vi "SubVI_Amplifier_Setup_Impedances.vi"(8 "error in (no error)":errorcluster, 9 "LINX Resource in":T1, 10 "Command Row Lenghts":u8[](array[numeric]), 11 "Amplifier Commands":u8[][](array[numeric])) -> (0 "error out":errorcluster, 3 "LINX Resource out":T1)   [LabVIEW 2020]
uses:
  <vilib>/MakerHub/LINX/Private/Type Defs/LINX Ref.ctl
  <vilib>/MakerHub/LINX/Private/Type Defs/Platform.ctl
  <vilib>/MakerHub/LINX/Private/Type Defs/Interface.ctl
  <vilib>/MakerHub/LINX/Private/Device/Type Defs/LINX Device Config.ctl
  <vilib>/MakerHub/LINX/Private/Device/Type Defs/TCP Config.ctl
  <vilib>/MakerHub/LINX/Private/Device/Type Defs/Channels.ctl
  <vilib>/MakerHub/LINX/Private/Type Defs/Peripherals/SPI/SPI Configuration.ctl
  <vilib>/MakerHub/LINX/Private/Type Defs/Peripherals/SPI/SPI Bit Order.ctl
  <vilib>/MakerHub/LINX/Private/Type Defs/Peripherals/SPI/SPI Mode.ctl
  <vilib>/MakerHub/LINX/Public/Peripherals/SPI/SPI CS Config.ctl
  <vilib>/MakerHub/LINX/Private/Type Defs/Peripherals/SPI/SPI CS Logic Level.ctl
  <vilib>/MakerHub/LINX/Public/Peripherals/Digital/Digital Write 1 Chan.vi
  <vilib>/MakerHub/LINX/Public/Peripherals/Digital/Digital Read 1 Chan.vi
  <vilib>/MakerHub/LINX/Public/Peripherals/SPI/SPI Write Read N Frames.vi
  <vilib>/MakerHub/LINX/Public/Peripherals/Digital/Digital Write N Chans.vi
  <vilib>/MakerHub/LINX/Public/Peripherals/Digital/Digital Read N Chans.vi
  <vilib>/MakerHub/LINX/Private/Local IO/LinxSpiWriteRead.vi
  <vilib>/MakerHub/LINX/Public/Utilities/Check Channel.vi
  <vilib>/MakerHub/LINX/Private/Local IO/LinxDigitalWrite.vi
  <vilib>/MakerHub/LINX/Private/Local IO/LinxDigitalRead.vi
  <vilib>/MakerHub/LINX/Private/Local IO/Handle Errors.vi
  <vilib>/MakerHub/LINX/Private/Utilties/Generate Error.vi
  Global 1.vi
  <vilib>/MakerHub/LINX/LMH-LINX.lvlib
  <vilib>/MakerHub/LINX/Private/Device/Device.lvlib
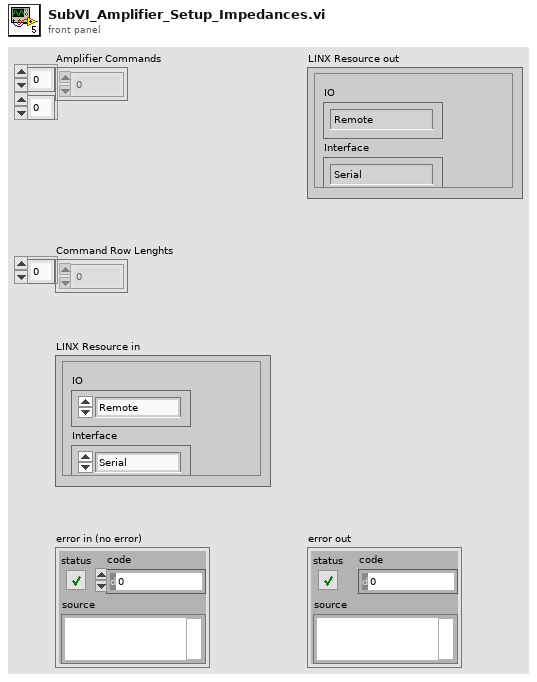
[diagram p1: front panel]
types:
  T1 = typedef "LMH-LINX.lvlib/LINX Ref.ctl" = cluster{"IO":T2, "Interface":T3, "LINX Device Config":T4}
  T2 = typedef "LMH-LINX.lvlib/Platform.ctl" = enum16{"Remote", "Local"}
  T3 = typedef "LMH-LINX.lvlib/Interface.ctl" = enum16{"Serial", "TCP"}
  T4 = typedef "LMH-LINX.lvlib/Device.lvlib/LINX Device Config.ctl" = cluster{"Interface":T3, "COM Port":refnum<visa-resource-name>, "TCP Configuration":T5, "Device Family":u8, "Device ID":u8, "Device Name":string, "TCP Ref":refnum<k5>, "Channels":T6}
  T5 = typedef "LMH-LINX.lvlib/Device.lvlib/TCP Config.ctl" = cluster{"IP Address":string, "Port":u16}
  T6 = typedef "LMH-LINX.lvlib/Channels.ctl" = cluster{"DI":u8[], "DO":u8[], "AI":u8[], "AO":u8[], "PWM":u8[], "QE":u8[], "UART":u8[], "I2C 2":u8[], "SPI":u8[], "CAN":u8[], "Servo":u8[], "AI Ref (V)":dbl, "AI Resolution (Bits)":u8, "AO Ref (V)":dbl, "AO Resolution (Bits)":u8}
  T7 = typedef "LMH-LINX.lvlib/SPI CS Config.ctl" = cluster{"CS Channel":u8, "CS Logic Level":T8}
  T8 = typedef "LMH-LINX.lvlib/SPI CS Logic Level.ctl" = enum8{"Active Low", "Active High"}
  T9 = typedef "LMH-LINX.lvlib/SPI Configuration.ctl" = cluster{"Clock Frequency":u32, "Bit Order":T10, "SPI Mode":T11}
  T10 = typedef "LMH-LINX.lvlib/SPI Bit Order.ctl" = enum8{"LSb First", "MSb First"}
  T11 = typedef "LMH-LINX.lvlib/SPI Mode.ctl" = enum8{"Mode 0", "Mode 1", "Mode 2", "Mode 3"}
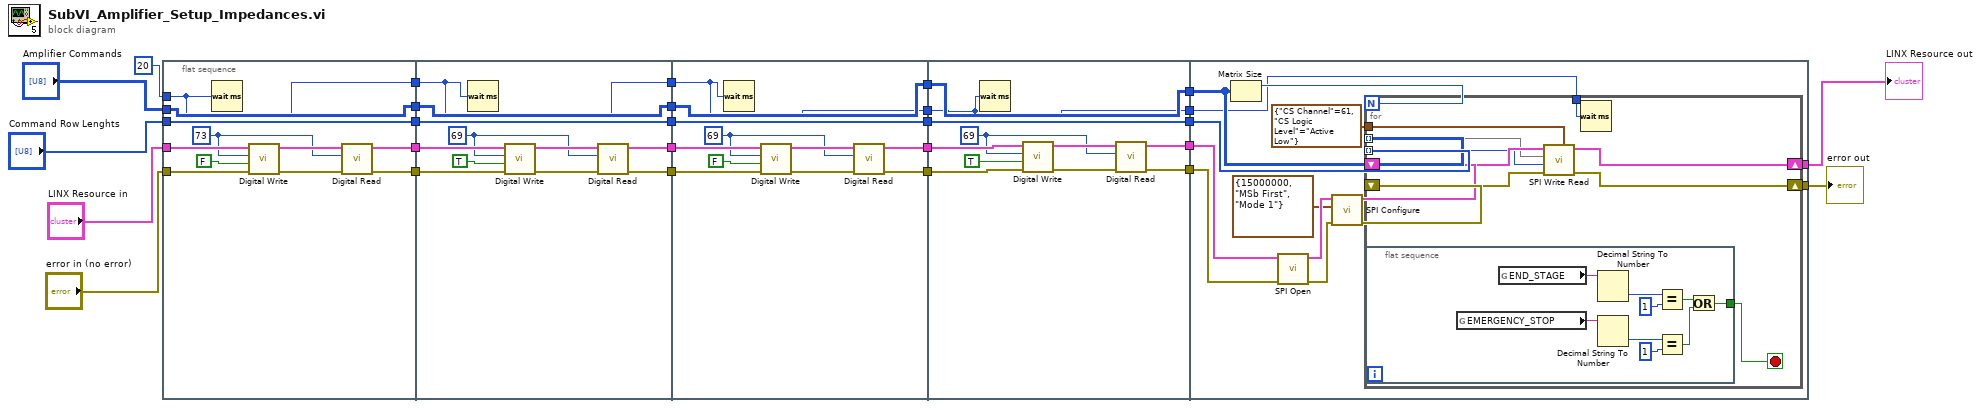
[diagram p0: block diagram]
diagram:
  n1 = flat-sequence {
    tunnel: "error in (no error)" -> [w37]
    tunnel: "LINX Resource in" -> [w36]
    tunnel: "Amplifier Commands" -> [w30]
    tunnel: "Command Row Lenghts" -> [w29]
    tunnel: [w30] -> w21
    tunnel: [w29] -> w20
    tunnel: [w32] -> w19
    tunnel: [w34] -> w18
    tunnel: u32 20 ("milliseconds to wait") -> [w28]
    tunnel: [w28] -> w4
    tunnel: w21 -> [w41]
    tunnel: w20 -> [w40]
    tunnel: w19 -> [w49]
    tunnel: w18 -> [w48]
    tunnel: [w41] -> w17
    tunnel: [w40] -> w16
    tunnel: [w43] -> w15
    tunnel: [w45] -> w14
    tunnel: w4 -> [w39]
    tunnel: [w39] -> w3
    tunnel: w17 -> [w52]
    tunnel: w16 -> [w51]
    tunnel: w15 -> [w59]
    tunnel: w14 -> [w58]
    tunnel: [w52] -> w13
    tunnel: [w51] -> w12
    tunnel: [w55] -> w11
    tunnel: [w54] -> w10
    tunnel: w3 -> [w50]
    tunnel: [w50] -> w2
    tunnel: w13 -> [w63]
    tunnel: w12 -> [w62]
    tunnel: w11 -> [w70]
    tunnel: w10 -> [w69]
    tunnel: [w63] -> w9
    tunnel: [w62] -> w8
    tunnel: [w65] -> w7
    tunnel: [w67] -> w6
    tunnel: w2 -> [w61]
    tunnel: [w61] -> w1
    tunnel: [w73] -> w25
    tunnel: [w74] -> w26
    tunnel: w9 -> [w77]
    tunnel: w8 -> [w78]
    tunnel: w7 -> [w81]
    tunnel: w6 -> [w82]
    tunnel: w1 -> [w72]
    frame #0 {
      w31 = u8 73 ("DO Channel")
      n2 = Wait (ms)(milliseconds to wait=w28) -> ()  [unwired: 1 out]
      n3 = call-poly <vilib>:"Digital Write.vi"("Error In"=w37, "Output Value"=FALSE, "DO Channel"=w31, "LINX Resource"=w36) -> ("Error Out"=w35:errorcluster, "LINX Resource"=w33:T1)  [unwired: 6 in]
      n4 = call-poly <vilib>:"Digital Read.vi"("Error In"=w35, "DI Channel"=w31, "LINX Resource"=w33) -> ("Error Out"=w34:errorcluster, "LINX Resource"=w32:T1)  [unwired: 6 in, 1 out]
    }
    frame #1 {
      w42 = u8 69 ("DO Channel")
      n5 = Wait (ms)(milliseconds to wait=w39) -> ()  [unwired: 1 out]
      n6 = call-poly <vilib>:"Digital Write.vi"("Error In"=w48, "Output Value"=TRUE, "DO Channel"=w42, "LINX Resource"=w49) -> ("Error Out"=w46:errorcluster, "LINX Resource"=w44:T1)  [unwired: 6 in]
      n7 = call-poly <vilib>:"Digital Read.vi"("Error In"=w46, "DI Channel"=w42, "LINX Resource"=w44) -> ("Error Out"=w45:errorcluster, "LINX Resource"=w43:T1)  [unwired: 6 in, 1 out]
    }
    frame #2 {
      w53 = u8 69 ("DO Channel")
      n8 = Wait (ms)(milliseconds to wait=w50) -> ()  [unwired: 1 out]
      n9 = call-poly <vilib>:"Digital Write.vi"("Error In"=w58, "Output Value"=FALSE, "DO Channel"=w53, "LINX Resource"=w59) -> ("Error Out"=w57:errorcluster, "LINX Resource"=w56:T1)  [unwired: 6 in]
      n10 = call-poly <vilib>:"Digital Read.vi"("Error In"=w57, "DI Channel"=w53, "LINX Resource"=w56) -> ("Error Out"=w54:errorcluster, "LINX Resource"=w55:T1)  [unwired: 6 in, 1 out]
    }
    frame #3 {
      w64 = u8 69 ("DO Channel")
      n11 = Wait (ms)(milliseconds to wait=w61) -> ()  [unwired: 1 out]
      n12 = call-poly <vilib>:"Digital Write.vi"("Error In"=w69, "Output Value"=TRUE, "DO Channel"=w64, "LINX Resource"=w70) -> ("Error Out"=w68:errorcluster, "LINX Resource"=w66:T1)  [unwired: 6 in]
      n13 = call-poly <vilib>:"Digital Read.vi"("Error In"=w68, "DI Channel"=w64, "LINX Resource"=w66) -> ("Error Out"=w67:errorcluster, "LINX Resource"=w65:T1)  [unwired: 6 in, 1 out]
    }
    frame #4 {
      n14 = Matrix Size(0:w77) -> (1:w80:i32)  [unwired: 1 out]
      n15 = call <vilib>:"SPI Open.vi"("Error In"=w82, "LINX Resource"=w81) -> ("Error Out"=w84:errorcluster, "LINX Resource"=w85:T1)  [unwired: 8 in]
      n16 = call <vilib>:"SPI Configure.vi"("Error In"=w84, "SPI Configuration"=T9 {"Clock Frequency"=15000000, "Bit Order"=enum."MSb First", "SPI Mode"=enum."Mode 1"}, "LINX Resource"=w85) -> ("Error Out"=w76:errorcluster, "LINX Resource"=w75:T1)  [unwired: 6 in, 1 out]
      n17 = for {
        N: w80 -> [_]
        shift-right: [w92] -> w74
        shift-left: w75 -> [w94]
        shift-right: [w91] -> w73
        shift-left: w76 -> [w93]
        tunnel: T7 {"CS Channel"=61, "CS Logic Level"=enum."Active Low"} ("CS Configuration") -> [w90]
        tunnel: w77 -> [w89] mode=indexing
        tunnel: w78 -> [w88] mode=indexing
        tunnel: w72 -> [w87]
        stop <- w86 stop-if-true
        n18 = flat-sequence {
          tunnel: [w95] -> w86
          frame #0 {
            n19 = global read "Global 1.vi" "EMERGENCY_STOP"() -> (w98:string)
            n20 = global read "Global 1.vi" "END_STAGE"() -> (w103:string)
            n21 = Decimal String To Number(string=w103) -> (number=w102:i32)  [unwired: 2 in, 1 out]
            n22 = Decimal String To Number(string=w98) -> (number=w100:i32)  [unwired: 2 in, 1 out]
            n23 = Equal?(x=w102, y=1) -> (x = y?=w96:bool)
            n24 = Equal?(x=w100, y=1) -> (x = y?=w97:bool)
            n25 = Or(x=w96, y=w97) -> (x .or. y?=w95:bool)
          }
        }
        n26 = call-poly <vilib>:"SPI Write Read.vi"("CS Configuration"=w90, "Error In"=w93, "SPI Frame Size"=w88, "Data"=w89, "LINX Resource"=w94) -> ("Error Out"=w91:errorcluster, "LINX Resource"=w92:T1)  [unwired: 3 in, 2 out]
        n27 = Wait (ms)(milliseconds to wait=w87) -> ()  [unwired: 1 out]
      }
    }
  }
  "LINX Resource out" <- w26
  "error out" <- w25
